vi "GetParameterList.vi"(8 "error in (no error)":errorcluster, 11 "HamaCam in":refnum<class "HamaCam.lvclass">) -> (0 "error out":errorcluster, 3 "HamaCam out":refnum<class "HamaCam.lvclass">)   [LabVIEW 2023, in "HamaCam.lvlib" / "HamaCam.lvclass"]
uses:
  HamaCam.lvclass
  HamaCam.lvclass/HamaCam.ctl
panel:
  out "Function List":T1(array[cluster])
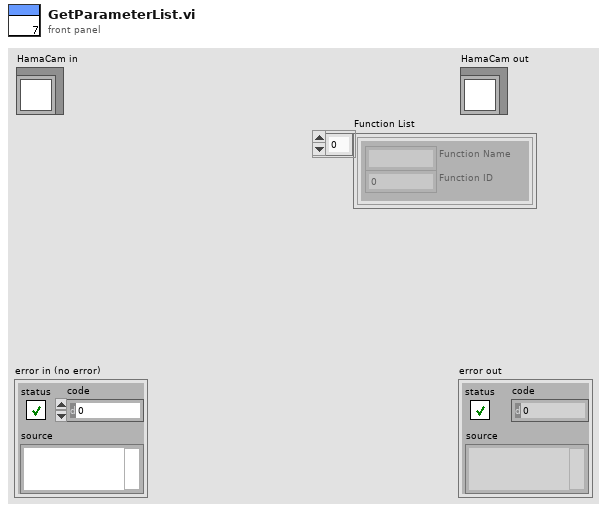
[diagram p1: front panel]
types:
  T1 = cluster{"Function Name":string, "Function ID":u32}[]
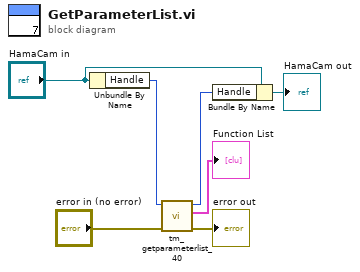
[diagram p0: block diagram]
diagram:
  n1 = Unbundle By Name("HamaCam in") -> ("Handle"=w6:u32)
  n2 = call "tm_getparameterlist_40.vi"("error in (no error)"="error in (no error)", "Handle in"=w6) -> ("error out"=→"error out":errorcluster, "Function List"=→"Function List":T1, "Handle out"=w3:u32)  [unwired: 7 in]
  n3 = Bundle By Name(cluster="HamaCam in", "Handle"=w3) -> (→"HamaCam out":refnum<class "HamaCam.lvclass">)
